vi "Picolog Temperature Array to Waveform.vi"(6 "Start Time":timestamp, 8 "Error In":errorcluster, 9 "Temperatures":sgl[][](array[numeric]), 10 "Times [s]":dbl[][](array[numeric])) -> (0 "Error Out":errorcluster, 1 "Temperature Waveforms":waveform(dbl)[](array[waveform]))   [LabVIEW 2017]
uses:
  <vilib>/Analysis/baseanly.llb/Mean (DBL).vi
  <vilib>/Analysis/NI_AALBase.lvlib
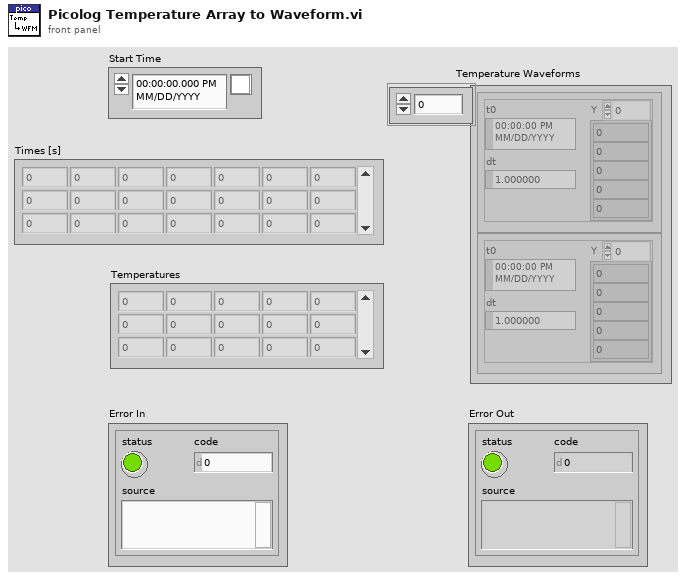
[diagram p1: front panel]
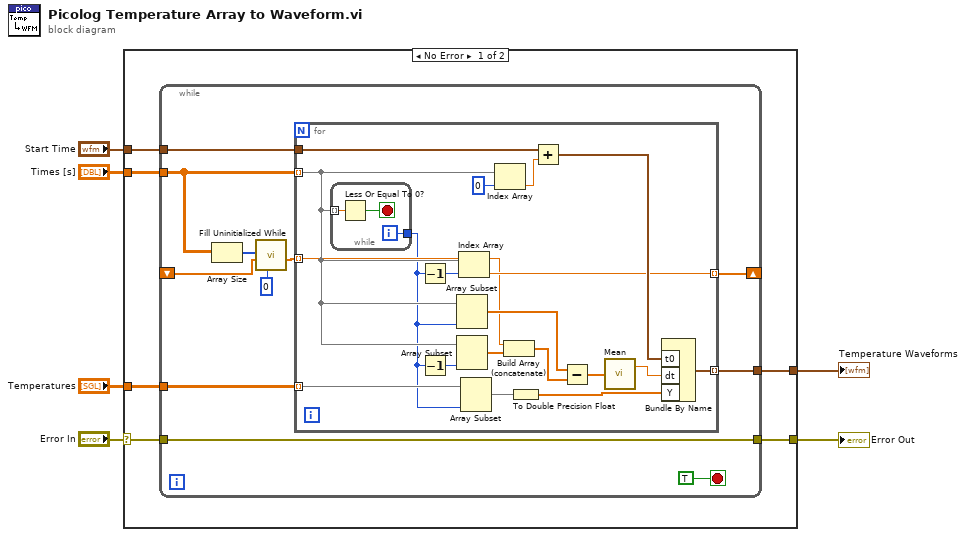
[diagram p0: block diagram]
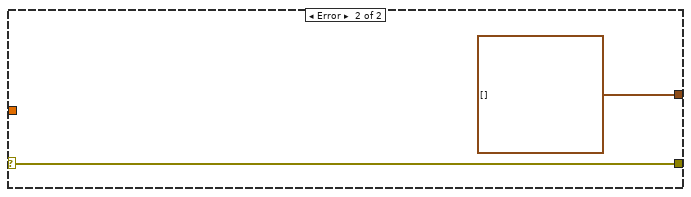
[diagram p2: hidden frame]
diagram:
  n1 = case shown="No Error" "Error In" {
    selector: "Error In" -> [w7 w47]
    tunnel: "Temperatures" -> [w12 _]
    tunnel: "Times [s]" -> [w11 _]
    tunnel: "Start Time" -> [w10 _]
    tunnel: [w9 w47] -> w3
    tunnel: [w8 waveform(sgl)[] [] ("Array")] -> w2
    frame No Error {
      n2 = while {
        tunnel: w12 -> [w23]
        tunnel: w11 -> [w17]
        tunnel: w10 -> [w22]
        tunnel: [w21] -> w8
        tunnel: w7 -> [w16]
        tunnel: [w16] -> w9
        shift-right: [w19] -> _
        shift-left: _ -> [w18]
        stop <- TRUE stop-if-true
        n3 = Array Size(array=w17) -> (size(s)=w14:i32[])
        n4 = call "Fill Uninitialized While.vi"("Dimension to check"=0, "Ref Array"=w18, "Data Array Size"=w14) -> ("Ref Array out"=w15:dbl[])  [unwired: 7 in, 1 out]
        n5 = for {
          tunnel: w23 -> [w42] mode=indexing
          tunnel: w22 -> [w37]
          tunnel: [w34] -> w21 mode=indexing
          tunnel: w17 -> [w28] mode=indexing
          tunnel: [w31] -> w19 mode=indexing
          tunnel: w15 -> [w30] mode=indexing
          n6 = while {
            tunnel: w28 -> [w45] mode=indexing
            tunnel: [w43] -> w26
            i -> [w43]
            stop <- w44 stop-if-true
            n7 = Less Or Equal To 0?(x=w45) -> (x <= 0?=w44:bool)
          }
          n8 = Decrement(x=w26) -> (x-1=w32:i32)
          n9 = Decrement(x=w26) -> (x-1=w27:i32)
          n10 = Array Subset(array=w28, length=w26) -> (w33:dbl[])  [unwired: 1 in]
          n11 = Array Subset(array=w28, length=w27) -> (w25:dbl[])  [unwired: 1 in]
          n12 = Index Array(array=w28, index=w32) -> (element=w31:dbl)
          n13 = Array Subset(array=w42, length=w26) -> (w41:sgl[])  [unwired: 1 in]
          n14 = Index Array(array=w28, index=0) -> (element=w36:dbl)
          n15 = Build Array (concatenate)(w30, w25) -> (w29:dbl[])
          n16 = To Double Precision Float(number=w41) -> (double precision float=w24:dbl[])
          n17 = Add(x=w37, y=w36) -> (x+y=w35:timestamp)
          n18 = Subtract(x=w33, y=w29) -> (x-y=w40:dbl[])
          n19 = call-poly <vilib>:"Mean.vi"("X"=w40) -> ("mean"=w39:dbl)  [unwired: 1 out]
          n20 = Bundle By Name("t0"=w35, "dt"=w39, "Y"=w24) -> (w34:waveform(dbl))  [unwired: 1 in]
        }
      }
    }
    frame Error {
    }
  }
  "Error Out" <- w3
  "Temperature Waveforms" <- w2
